vi "insertTubelwithTimeStamp.vi"(8 "error in (no error)":errorcluster, 10 "Name of Table":string, 11 "DataCollector in":refnum<class "DataCollector.lvclass">) -> (0 "error out":errorcluster, 3 "DataCollector out":refnum<class "DataCollector.lvclass">)   [LabVIEW 2017, in "DataCollector.lvclass"]
uses:
  DataCollector.lvclass
  DataCollector.lvclass/DataCollector.ctl
  <vilib>/drjdpowell/SQLite Library/SQL Statement/SQL Statement.lvclass/SQL Statement.ctl
  <vilib>/drjdpowell/SQLite Library/SQL Statement/Bind Null.vi
  <vilib>/drjdpowell/SQLite Library/SQL Statement/Bind Integer.vi
  <vilib>/drjdpowell/SQLite Library/SQL Statement/Step.vi
  <vilib>/drjdpowell/SQLite Library/SQL Statement/Error Message.vi
  <vilib>/drjdpowell/SQLite Library/SQL Connection/Connection.lvclass
  <vilib>/drjdpowell/SQLite Library/SQL Statement/SQL Statement.lvclass
  <vilib>/drjdpowell/SQLite Library/Transaction Helpers/Transaction.lvlib
panel:
  out "concatenated string":string
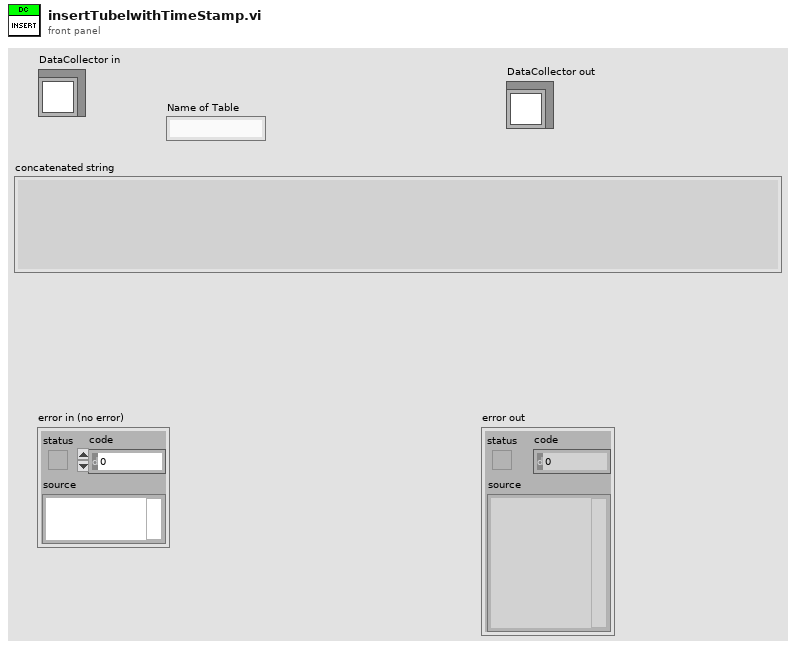
[diagram p1: front panel]
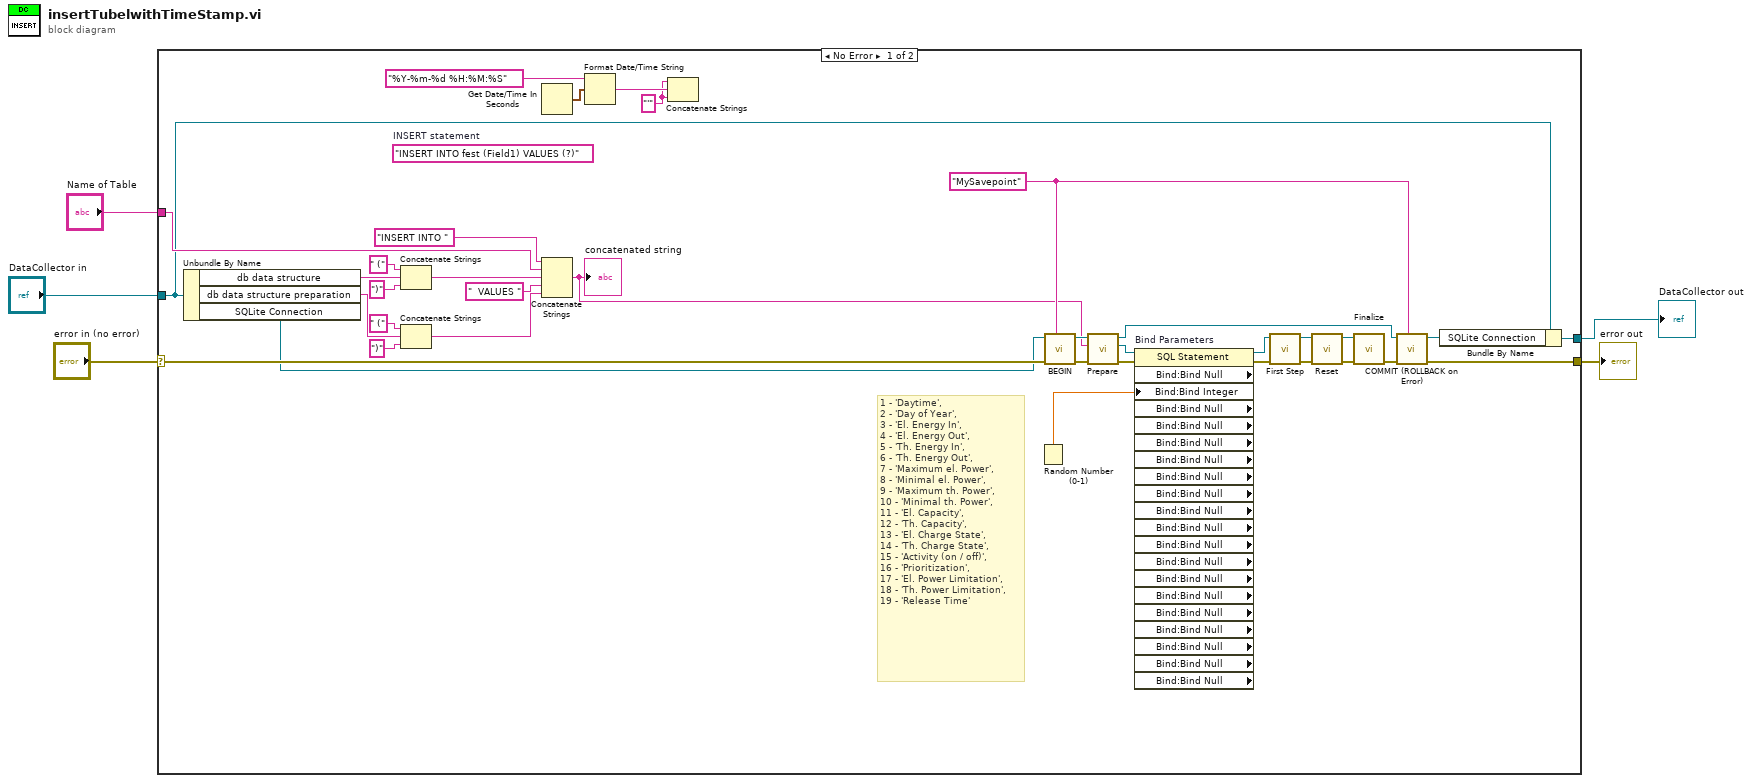
[diagram p0: block diagram]
diagram:
  n1 = case shown="No Error" "error in (no error)" {
    selector: "error in (no error)" -> [w13 w43]
    tunnel: [w12 w43] -> w3
    tunnel: [w14 w42] -> w5
    tunnel: "DataCollector in" -> [w6 w42]
    tunnel: "Name of Table" -> [w25 _]
    frame No Error {
      (unwired) "INSERT INTO fest (Field1) VALUES (?)"  # INSERT statement
      w11 = "MySavepoint" ("Savepoint name")
      w40 = "'" ("String")
      # "1 - 'Daytime', \n2 - 'Day of Year', \n3 - 'El. Energy In',  \n4 - 'El. Energy Out', \n5 - 'Th. Energy In',  \n6 - 'Th. Energy Out',  \n7 - 'Maximum el. Power', \n8 - 'Minimal el. Power', \n9 - 'Maximum th. Power', \n10 - 'Minimal th. Power', \n11 - 'El. Capacity',  \n12 - 'Th. Capacity',\n13 - 'El. Charge State', \n14 - 'Th. Charge State', \n15 - 'Activity (on / off)', \n16 - 'Prioritization', \n17 - 'El. Power Limitation',  \n18 - 'Th. Power Limitation',\n19 - 'Release Time'"
      n2 = Unbundle By Name(w6) -> ("db data structure"=w21:string, "db data structure preparation"=w17:string, "SQLite Connection"=w9:refnum<class "Connection.lvclass">)
      n3 = Concatenate Strings(" (" ("string"), w21, ")" ("string")) -> (w20:string)
      n4 = Concatenate Strings(" (" ("string"), w17, ")" ("string")) -> (w16:string)
      n5 = Get Date/Time In Seconds() -> (seconds since 1Jan1904=w10:timestamp)
      n6 = Concatenate Strings("INSERT INTO " ("string"), w25, w20, "  VALUES " ("string"), w16) -> (w8:string)
      "concatenated string" <- w8
      n7 = Format Date/Time String(time format string (%c)="%Y-%m-%d %H:%M:%S" ("Zeitformatierungs-String (%c)"), seconds (now)=w10) -> (date/time string=w41:string)  [unwired: 1 in]
      n8 = Concatenate Strings(w40, w41, w40) -> ()  [unwired: 1 out]
      n9 = Random Number (0-1)() -> (number: 0 to 1=w7:dbl)
      n10 = call <vilib>:"BEGIN.vi"("Savepoint name"=w11, "error in (no error)"=w13, "Connection in"=w9) -> ("error out"=w36:errorcluster, "Connection out"=w35:refnum<class "Connection.lvclass">)  [unwired: 7 in]
      n11 = call <vilib>:"Prepare.vi"("error in (no error)"=w36, "SQL"=w8, "SQLite Connection in"=w35) -> ("error out"=w32:errorcluster, "SQL Statement out"=w31:refnum<class "SQL Statement.lvclass">, "SQLite Connection out"=w37:refnum<class "Connection.lvclass">)  [unwired: 4 in, 2 out]
      n12 = property on="Bind Parameters" class="SQL Statement" props=["Bind:Bind Null", "Bind:Bind Integer", "Bind:Bind Null", "Bind:Bind Null", "Bind:Bind Null", "Bind:Bind Null", "Bind:Bind Null", "Bind:Bind Null", "Bind:Bind Null", "Bind:Bind Null", "Bind:Bind Null", "Bind:Bind Null", "Bind:Bind Null", "Bind:Bind Null", "Bind:Bind Null", "Bind:Bind Null", "Bind:Bind Null", "Bind:Bind Null", "Bind:Bind Null"](reference=w31, error in=w32, "Bind:Bind Integer"=w7) -> (reference out=w30:refnum<class "SQL Statement.lvclass">, error out=w29:errorcluster)  [unwired: 18 out]
      n13 = call <vilib>:"First Step.vi"("error in (no error)"=w29, "SQL Statement in"=w30) -> ("error out"=w28:errorcluster, "SQL Statement out"=w27:refnum<class "SQL Statement.lvclass">)  [unwired: 7 in, 1 out]
      n14 = call <vilib>:"Reset.vi"("error in (no error)"=w28, "SQL Statement in"=w27) -> ("error out"=w34:errorcluster, "SQL Statement out"=w33:refnum<class "SQL Statement.lvclass">)  [unwired: 8 in]
      n15 = call <vilib>:"Finalize.vi"("error in (no error)"=w34, "SQL Statement in"=w33) -> ("error out"=w38:errorcluster)  [unwired: 9 in]
      n16 = call <vilib>:"COMMIT (ROLLBACK on Error).vi"("Savepoint name"=w11, "error in (no error)"=w38, "Connection in"=w37) -> ("error out"=w12:errorcluster, "Connection out"=w15:refnum<class "Connection.lvclass">)  [unwired: 7 in]
      n17 = Bundle By Name(cluster=w6, "SQLite Connection"=w15) -> (w14:refnum<class "DataCollector.lvclass">)
    }
    frame Error {
    }
  }
  "error out" <- w3
  "DataCollector out" <- w5
